vi "Point_Read.vi"   [LabVIEW 2017, in "PointValueMap.lvlib"]
doc: "Gets the value of a map point."
uses:
  <vilib>/addons/PointValueMap/PointValueMap.lvlib
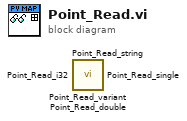
[diagram p0: block diagram]
diagram:
  n1 = call <vilib>:"Point_Read_variant.vi"() -> ()  [unwired: 6 in, 6 out]
  n2 = call <vilib>:"Point_Read_string.vi"() -> ()  [unwired: 6 in, 6 out]
  n3 = call <vilib>:"Point_Read_i32.vi"() -> ()  [unwired: 6 in, 6 out]
  n4 = call <vilib>:"Point_Read_single.vi"() -> ()  [unwired: 6 in, 6 out]
  n5 = call <vilib>:"Point_Read_double.vi"() -> ()  [unwired: 6 in, 6 out]
